vi "Close File.vi"(8 "error in (no error)":errorcluster, 11 "Refnum out":refnum<k34>) -> (0 "error out":errorcluster)   [LabVIEW 2019, in "FileReader.lvlib"]
doc: "This VI closes the current Log File.\n_____\nBased on DQMH Project Template 6.1.0.94."
uses:
  FileReader.lvlib
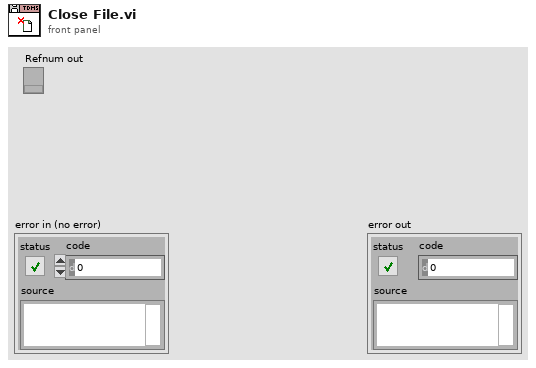
[diagram p1: front panel]
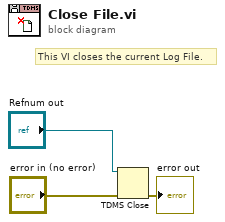
[diagram p0: block diagram]
diagram:
  # "This VI closes the current Log File."
  n1 = TDMS Close(8:"error in (no error)", 11:"Refnum out") -> (0:→"error out":errorcluster)  [unwired: 1 out]
